vi "LVClass_CorrectionDataManager CheckRelativePositionsSaturation.vi"(0 "CorrectionDataManager in":refnum<class "CorrectionDataManager.lvclass">, 5 "Deltaposition":sgl[](array[numeric]), 7 "position":sgl[](array[numeric]), 11 "error in (no error)":errorcluster) -> (4 "CorrectionDataManager out":refnum<class "CorrectionDataManager.lvclass">, 10 "saturated_act_count":i32, 15 "error out":errorcluster)   [LabVIEW 2020, in "CorrectionDataManager.lvclass"]
doc: "Count the number of actuators which will be saturated (reaching min or max of\ntheir positions) if relative command is applied.\n\n<B>corrdata_managerIn</B> : WavefrontCorrector object.\n<B>corrdata_managerOut</B> : WavefrontCorrector object.\n<B>current_position</B> : Array of current wavefront corrector positions.\n<B>delta_commands</B> : Array of delta commands.\n<B>saturated_act_count</B> : Count of actuators which will be at min or max of their positions if command\n is applied."
uses:
  CorrectionDataManager.lvclass
  CorrectionDataManager.lvclass/CorrectionDataManager.ctl
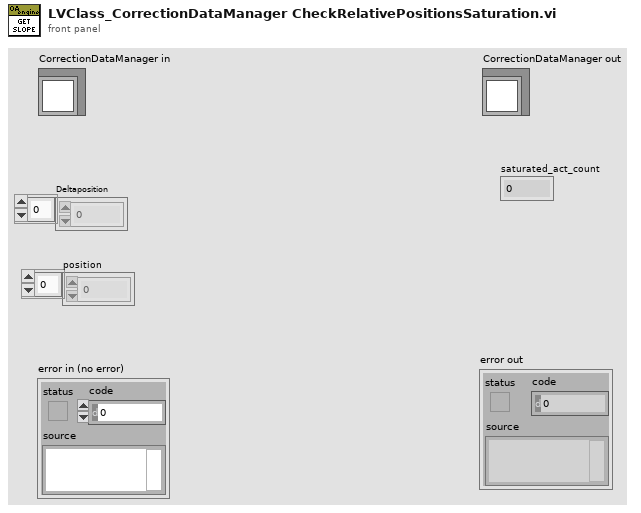
[diagram p1: front panel]
types:
  T1 = typedef "ClassID.ctl" = i64
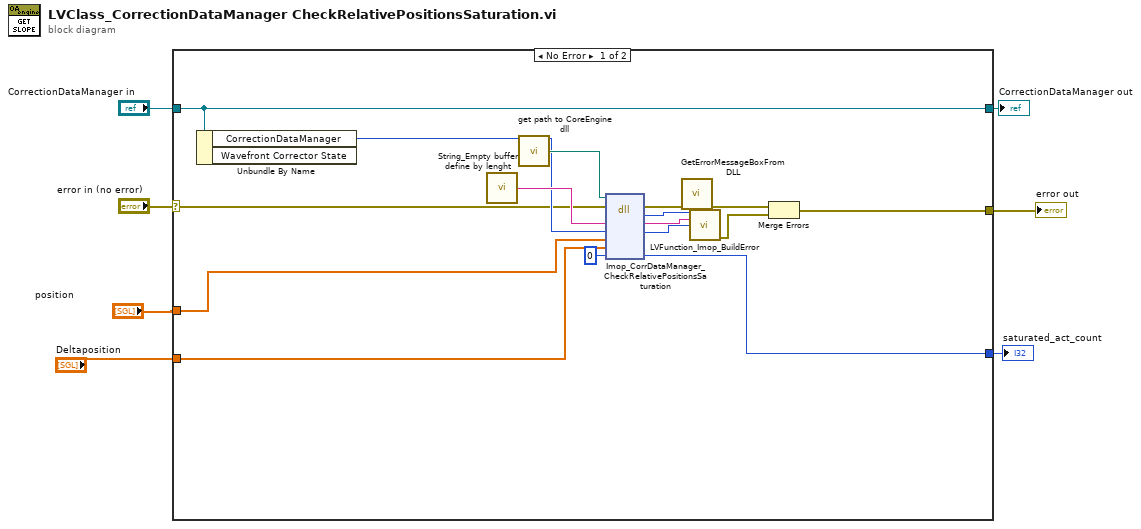
[diagram p0: block diagram]
diagram:
  n1 = case shown="No Error" "error in (no error)" {
    selector: "error in (no error)" -> [w13 w25]
    tunnel: [w21 w25] -> w5
    tunnel: [w20 w24] -> w4
    tunnel: "CorrectionDataManager in" -> [w20 w24]
    tunnel: "position" -> [w12 _]
    tunnel: [w9 _] -> w1
    tunnel: "Deltaposition" -> [w11 _]
    frame No Error {
      n2 = Unbundle By Name(w20) -> ("CorrectionDataManager"=w14:T1)  [unwired: 1 out]
      n3 = call "String_Empty buffer define by lenght.vi"() -> ("Empty buffer"=w18:string)  [unwired: 1 in]
      n4 = call "get path to CoreEngine dll.vi"() -> ("path to wavekit library"=w19:path)  [unwired: 14 in, 1 out]
      n5 = dll-call lib="D:/soft/HASO_v3/SVN_trunk/ImOpCoreEngine4_LV2011/DLLs/c_interface_vc100.dll" fn="Imop_CorrDataManager_CheckRelativePositionsSaturation"(path in=w19, error in=w13, "message"=w18, "WavefrontCorrection"=w14, "current position"=w12, "delta position"=w11, "saturated_act_count"=0) -> (error out=w17:errorcluster, "return type"=w16:i32, "message"=w15:string, "WavefrontCorrection"=w8:i64, "saturated_act_count"=w9:i32)  [unwired: 3 in, 1 out]
      n6 = call "GetErrorMessageBoxFromDLL.vi"("error IN"=w17) -> ("error OUT"=w23:errorcluster)  [unwired: 10 in]
      n7 = call "LVFunction_Imop_BuildError.vi"("code"=w16, "String to Prepend to source (\"\")"=w15, "Adresse"=w8) -> ("error out"=w22:errorcluster)  [unwired: 12 in]
      n8 = Merge Errors(w23, w22) -> (w21:errorcluster)
    }
    frame Error {
    }
  }
  "error out" <- w5
  "CorrectionDataManager out" <- w4
  "saturated_act_count" <- w1
